vi "Setup.vi"(8 "Error In":errorcluster, 11 "String":string) -> (0 "Error Out":errorcluster, 3 "Lexer":refnum<class "Lexer.lvclass">)   [LabVIEW 2018, in "Tests.lvlib" / "Lexer.lvlib"]
uses:
  Lexer.lvlib
  src/Toolkit/Low-Level/Lexer/Lexer.lvclass
  src/Toolkit/Low-Level/Readers/String/String.lvclass
  D:/Users/cfield/Code/Field R&D Services/Labstache/src/Toolkit/Low-Level/Readers/Reader/Reader.lvclass
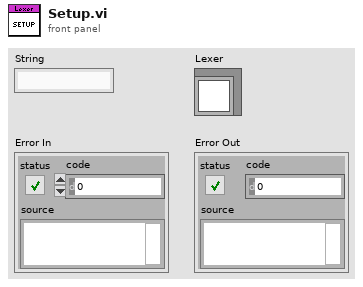
[diagram p1: front panel]
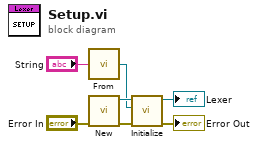
[diagram p0: block diagram]
diagram:
  n1 = call "From.vi"("Value"="String") -> ("String"=w1:refnum<class "String.lvclass">)
  n2 = call "New.vi"("Error In"="Error In") -> ("Error Out"=w2:errorcluster, "Lexer"=w3:refnum<class "Lexer.lvclass">)  [unwired: 9 in]
  n3 = call-dynamic "Initialize.vi"("Error In"=w2, "Reader"=w1, "Lexer In"=w3) -> ("Error Out"=→"Error Out":errorcluster, "Lexer Out"=→"Lexer":refnum<class "Lexer.lvclass">)  [unwired: 7 in]
